vi "testjson2.vi"() -> ()   [LabVIEW 2014]
uses:
  controls/Pajson.ctl
panel:
  out "value 2":T1(array[cluster])
  in  "Array":T1(array[cluster])
  out "JSON string":string
  out "value":T2
  in  "json":T3
  out "error out":errorcluster
  in  "error in":errorcluster
  out "text":string
  in  "Path":path
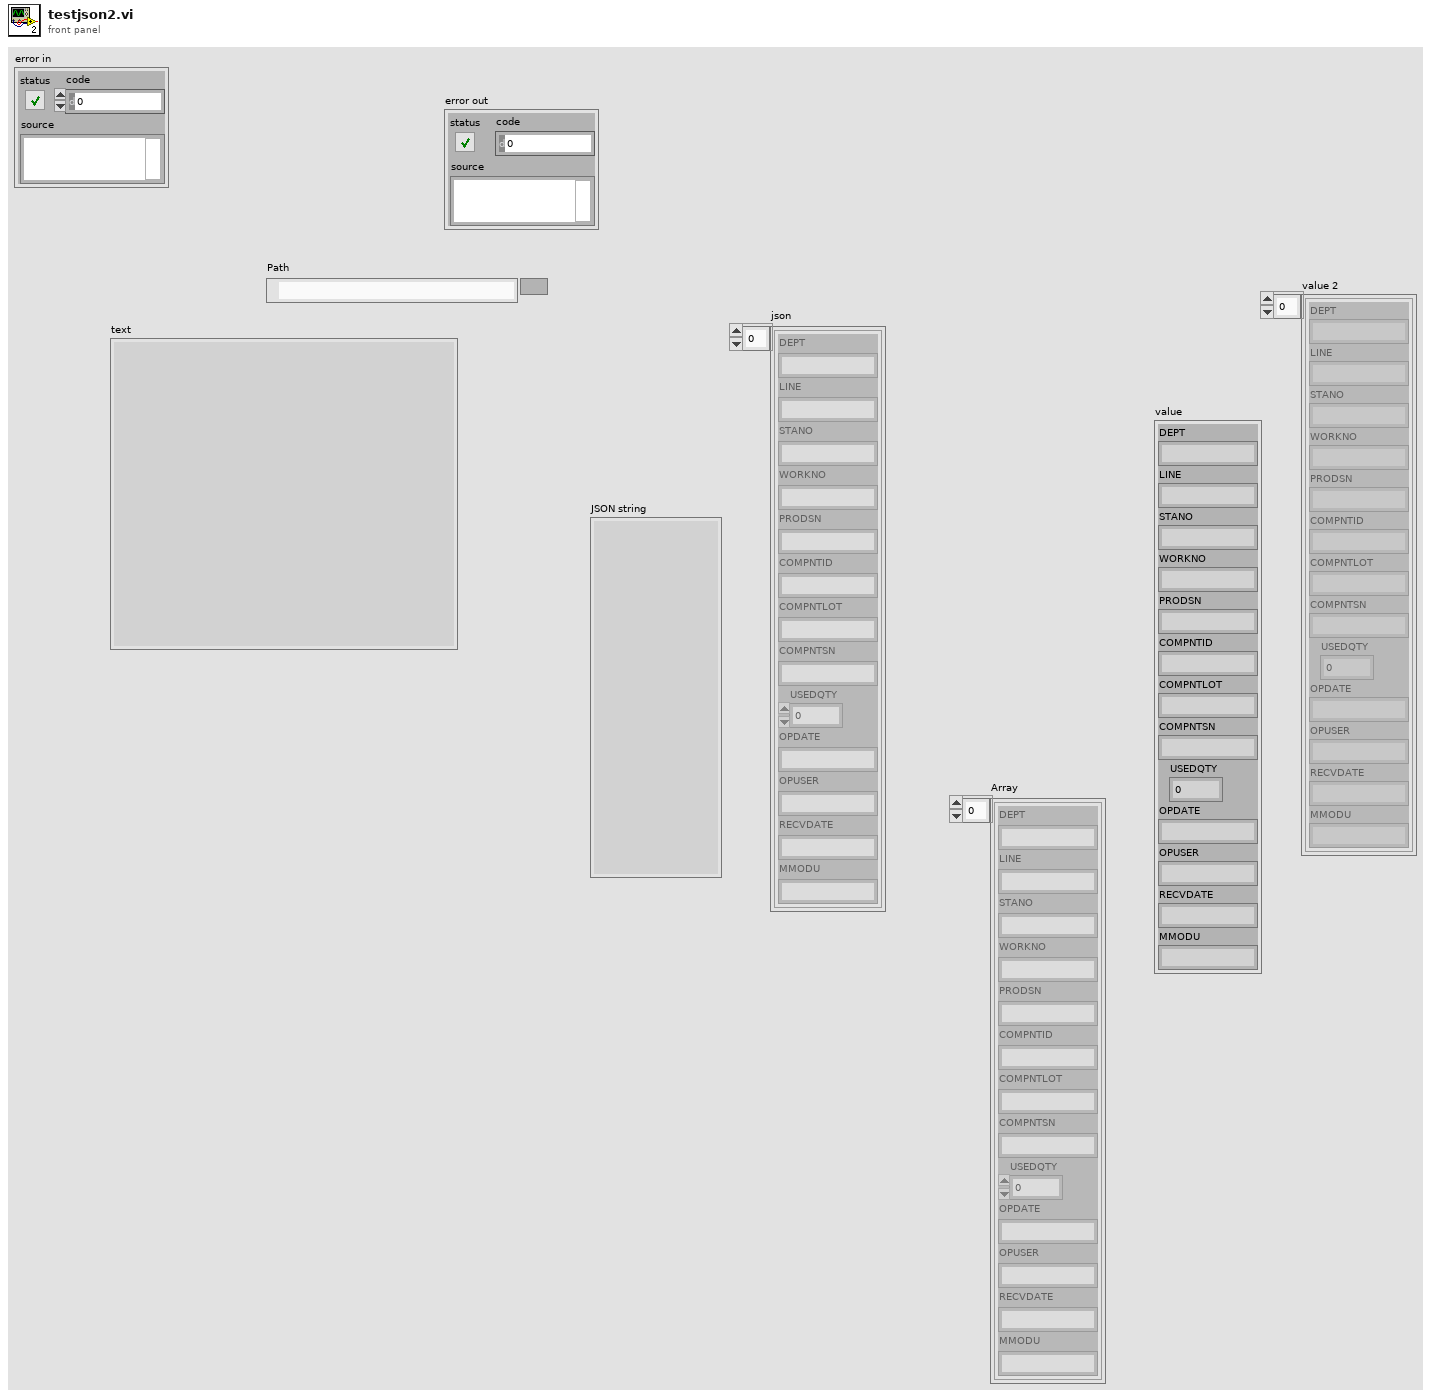
[diagram p1: front panel]
types:
  T1 = cluster{"DEPT":string, "LINE":string, "STANO":string, "WORKNO":string, "PRODSN":string, "COMPNTID":string, "COMPNTLOT":string, "COMPNTSN":string, "USEDQTY":i16, "OPDATE":string, "OPUSER":string, "RECVDATE":string, "MMODU":string}[]
  T2 = cluster{"DEPT":string, "LINE":string, "STANO":string, "WORKNO":string, "PRODSN":string, "COMPNTID":string, "COMPNTLOT":string, "COMPNTSN":string, "USEDQTY":i16, "OPDATE":string, "OPUSER":string, "RECVDATE":string, "MMODU":string}
  T3 = typedef "Pajson.ctl" = cluster{"DEPT":string, "LINE":string, "STANO":string, "WORKNO":string, "PRODSN":string, "COMPNTID":string, "COMPNTLOT":string, "COMPNTSN":string, "USEDQTY":i16, "OPDATE":string, "OPUSER":string, "RECVDATE":string, "MMODU":string}[]
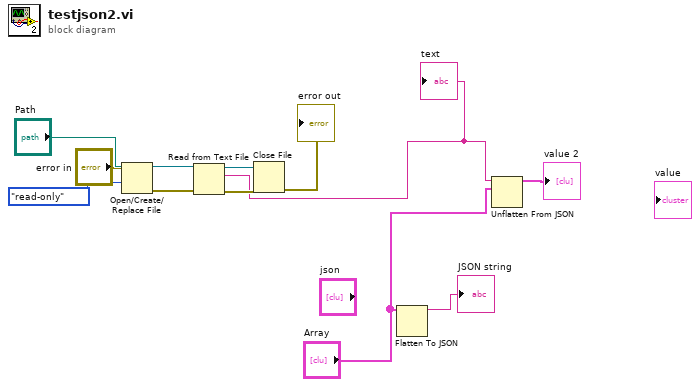
[diagram p0: block diagram]
diagram:
  n1 = Open/Create/Replace File(file path (use dialog)="Path", error in="error in", access (0:read/write)=enum16{"read/write", "read-only", "write-only"}."read-only") -> (refnum out=w11:refnum<file>, error out=w9:errorcluster)  [unwired: 3 in, 1 out]
  n2 = Read from Text File(file (use dialog)=w11, error in=w9) -> (refnum out=w10:refnum<file>, text=w3:string, error out=w8:errorcluster)  [unwired: 2 in, 1 out]
  "text" <- w3
  n3 = Close File(refnum=w10, error in=w8) -> (error out=→"error out":errorcluster)  [unwired: 1 out]
  n4 = Flatten To JSON(anything="Array") -> (JSON string=→"JSON string":string)  [unwired: 2 in, 1 out]
  n5 = Unflatten From JSON(JSON string=w3, type and defaults="Array") -> (value=→"value 2":T1)  [unwired: 5 in, 1 out]
